vi "Set Refresh Rate.vi"(8 "error in (no error)":errorcluster, 10 "Value":i32, 11 "Item Ref in":T1 format="%.0x") -> (0 "error out":errorcluster, 3 "Item Ref out":T1 format="%.0x")   [LabVIEW 2020, in "Modbus Master System Explorer.lvlib"]
uses:
  Modbus Master System Explorer.lvlib
  <vilib>/NI VeriStand/Custom Device API/Custom Device Item Ref.ctl
  Shared/Constants.vi
  <vilib>/NI VeriStand/Custom Device API/Set Item Property (I32).vi
  Shared/Modbus Master Shared.lvlib
  <vilib>/NI VeriStand/Custom Device API/Custom Device API.lvlib
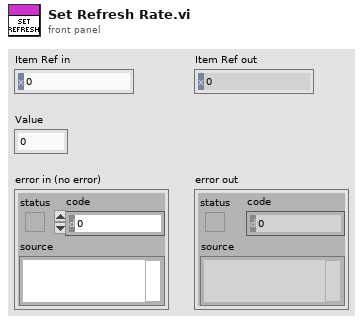
[diagram p1: front panel]
types:
  T1 = typedef "Custom Device API.lvlib/Custom Device Item Ref.ctl" = u64
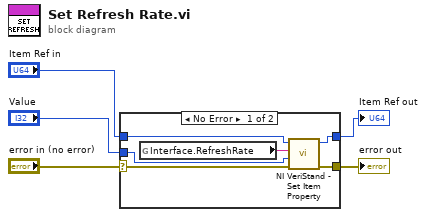
[diagram p0: block diagram]
diagram:
  n1 = case shown="No Error" "error in (no error)" {
    selector: "error in (no error)" -> [w10 w12]
    tunnel: "Value" -> [w9 _]
    tunnel: "Item Ref in" -> [w8 w13]
    tunnel: [w7 w12] -> w2
    tunnel: [w6 w13] -> w1
    frame No Error {
      n2 = global read "Constants.vi" "Interface.RefreshRate"() -> (w11:string)
      n3 = call-poly <vilib>:"NI VeriStand - Set Item Property.vi"("error in (no error)"=w10, "Value"=w9, "Property Name"=w11, "Item Ref in"=w8) -> ("error out"=w7:errorcluster, "Item Ref out"=w6:T1)  [unwired: 5 in, 1 out]
    }
    frame Error {
    }
  }
  "error out" <- w2
  "Item Ref out" <- w1
